vi "Get_Text_Argument.vi"(1 "Argument":string, 2 "Argument List":string[](array[string])) -> (0 "Text":string)   [LabVIEW 2011]
doc: "This VI parses an argument to find it's text value. For example, given an argument in the form of Arg(\"some text\"), it would return \"some text\", without quotation marks."
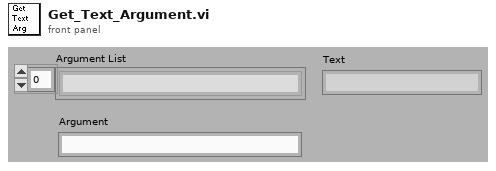
[diagram p1: front panel]
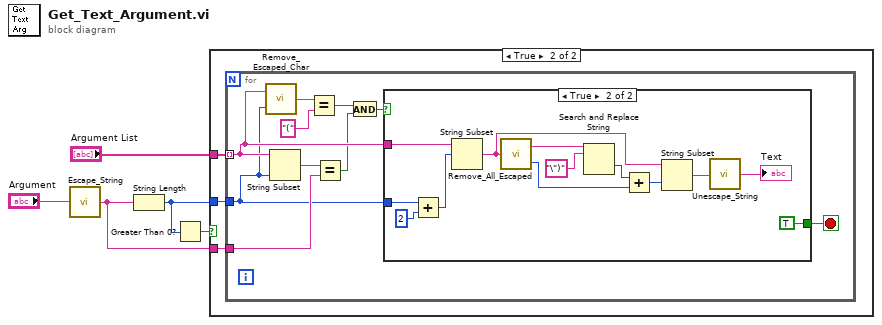
[diagram p0: block diagram]
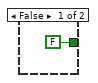
[diagram p3: hidden frame]
diagram:
  n1 = call "Escape_String.vi"("Input String"="Argument") -> ("Escaped String"=w3:string)
  n2 = String Length(string=w3) -> (length=w1:i32)
  n3 = Greater Than 0?(x=w1) -> (x > 0?=w2:bool)
  n4 = case shown="True" w2 {
    tunnel: "Argument List" -> [_ w8]
    tunnel: w1 -> [_ w7]
    tunnel: w3 -> [_ w6]
    frame False {
    }
    frame True {
      n5 = for {
        tunnel: w8 -> [w12] mode=indexing
        tunnel: w7 -> [w11]
        tunnel: w6 -> [w16]
        stop <- w17 stop-if-true
        n6 = call "Remove_Escaped_Char.vi"("Offset"=w11, "Input String"=w12) -> ("Output String"=w15:string)
        n7 = String Subset(string=w12, length (rest)=w11) -> (substring=w18:string)  [unwired: 1 out]
        n8 = Equal?(x=w15, y="(") -> (x = y?=w9:bool)
        n9 = Equal?(x=w18, y=w16) -> (x = y?=w10:bool)
        n10 = And(x=w9, y=w10) -> (x .and. y?=w13:bool)
        n11 = case shown="True" w13 {
          tunnel: w12 -> [_ w28]
          tunnel: [FALSE TRUE] -> w17
          tunnel: w11 -> [_ w26]
          frame False {
          }
          frame True {
            n12 = Add(x=w26, y=2) -> (x+y=w25:i32)
            n13 = String Subset(string=w28, offset (0)=w25) -> (substring=w27:string)  [unwired: 1 in]
            n14 = call "Remove_All_Escaped.vi"("Input String"=w27) -> ("Output String"=w30:string, "Chars Removed"=w23:i32)
            n15 = Search and Replace String(input string=w30, search string="\")") -> (offset past replacement=w22:i32)  [unwired: 6 in, 3 out]
            n16 = Add(x=w22, y=w23) -> (x+y=w21:i32)
            n17 = String Subset(string=w27, length (rest)=w21) -> (substring=w32:string)  [unwired: 1 in]
            n18 = call "Unescape_String.vi"("Input String"=w32) -> ("Output String"=→"Text":string)
          }
        }
      }
    }
  }
